vi "Periodic Tasks.vi"(8 "error in":errorcluster) -> ()   [LabVIEW 2019]
doc: "This VI runs in parallel to other tasks. It can contain as many user-defined periodic loops as you need. These can carry out PID or other sorts of timed response."
uses:
  <vilib>/Rock Robotics/WPI/Relay/WPI_RelayValue.ctl
  <vilib>/Rock Robotics/WPI/ThirdParty/Phoenix-LabVIEW/Motor Controller/Controls/CTRE_Phoenix_MotorControl_ControlMode.ctl
  <vilib>/Rock Robotics/WPI/Solenoid/WPI_SolenoidValue.ctl
  Driver Globals.vi
  <vilib>/Rock Robotics/WPI/Solenoid/WPI_SolenoidSetEnum.vi
panel:
  in  "Proportional":dbl
  in  "Integral":dbl
  in  "Derivative":dbl
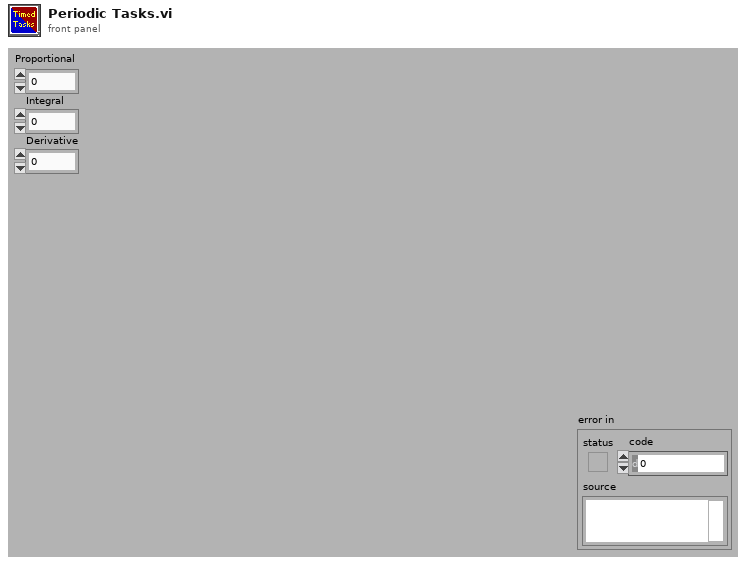
[diagram p1: front panel]
types:
  T1 = typedef "WPI_RelayValue.ctl" = enum16{"Off", "On", "Forward", "Reverse"}
  T2 = enum16{"DemandType_Neutral", "DemandType_AuxPID", "DemandType_ArbitraryFeedForward"}
  T3 = typedef "WPI_SolenoidValue.ctl" = enum16{"Off", "On", "Forward", "Reverse"}
  T4 = typedef "Color Sensor V3 DevRef.ctl" = cluster{"I2CDevRef":T5}
  T5 = typedef "WPI_I2CDevRef.ctl" = cluster{"DevStatus":errorcluster, "Device Address":u8, "Handle":i32, "I2C Bus":T6}
  T6 = typedef "i2c_bus.ctl" = enum16{"I2C On-Board", "I2C MXP", "Invalid"}
  T7 = typedef "WPI_EncoderDevRef.ctl" = cluster{"DevStatus":errorcluster, "EncoderIndex":T8, "CounterIndex":T9, "DistancePerCount":dbl, "Decoding Type":T10}
  T8 = typedef "FPGA_EncoderIdx.ctl" = enum8{"Enc 0", "Enc 1", "Enc 2", "Enc 3", "Enc 4", "Enc 5", "Enc 6", "Enc 7", "Invalid"}
  T9 = typedef "FPGA_CounterCtrSystemIndex.ctl" = enum8{"Ctr 0", "Ctr 1", "Ctr 2", "Ctr 3", "Ctr 4", "Ctr 5", "Ctr 6", "Ctr 7", "Invalid"}
  T10 = typedef "WPI_EncoderType.ctl" = enum16{"1x", "2x", "4x"}
  T11 = typedef "WPI_MotorControlDeviceRef.ctl" = cluster{"DeviceStatus":errorcluster, "Type":T12, "PWM":cluster{"PWM Channel":T13, "DeadBand":T14}, "CAN":cluster{"Device Number":u8, "SetOutput VI Ref":variant, "GetOutput VI Ref":variant, "Enable VI Ref":variant, "Disable VI Ref":variant, "Data":variant}, "Invert":bool, "DIO PWM":cluster{"PWM \"Enable\" Channel":T13, "DIOChannel":T15, "PWM Rate":dbl}}
  T12 = typedef "WPI_MotorControlType.ctl" = enum16{"PWM", "CAN", "DIO PWM"}
  T13 = typedef "FPGA_DIOPWMChannel.ctl" = enum8{"PWM 0", "PWM 1", "PWM 2", "PWM 3", "PWM 4", "PWM 5", "PWM 6", "PWM 7", "PWM 8", "PWM 9", "PWM MXP 0", "PWM MXP 1", "PWM MXP 2", "PWM MXP 3", "PWM MXP 4", "PWM MXP 5", "PWM MXP 6", "PWM MXP 7", "PWM MXP 8", "PWM MXP 9", "Invalid"}
  T14 = typedef "WPI_PWMDeadband.ctl" = cluster{"Name":string, "maxPositivePwm":i32, "minPositivePwm":i32, "centerPwm":i32, "maxNegativePwm":i32, "minNegativePwm":i32, "angularRange":u16}
  T15 = typedef "FPGA_DIOChannel.ctl" = enum8{"DIO 0", "DIO 1", "DIO 2", "DIO 3", "DIO 4", "DIO 5", "DIO 6", "DIO 7", "DIO 8", "DIO 9", "DIO MXP 0", "DIO MXP 1", "DIO MXP 2", "DIO MXP 3", "DIO MXP 4", "DIO MXP 5", "DIO MXP 6", "DIO MXP 7", "DIO MXP 8", "DIO MXP 9", "DIO MXP 10", "DIO MXP 11", "DIO MXP 12", "DIO MXP 13", "DIO MXP 14", "DIO MXP 15", "SPI Port CS1", "SPI Port CS2", "SPI Port CS3", "SPI Port MISO", "SPI Port MOSI", "Invalid"}
  T16 = typedef "WPI_AnalogChannelDevRef.ctl" = cluster{"DevStatus":errorcluster, "Analog Channel":T17}
  T17 = typedef "FPGA_AIChannel.ctl" = enum8{"AI 0", "AI 1", "AI 2", "AI 3", "AI MXP 0", "AI MXP 1", "AI MXP 2", "AI MXP 3", "Invalid"}
  T18 = typedef "WPI_SolenoidDevRef.ctl" = cluster{"DevStatus":errorcluster, "Pneumatics Control Module":u8, "Forward Solenoid Channel":T19, "Reverse Solenoid Channel":T19}
  T19 = typedef "WPI_SolenoidChannel.ctl" = enum8{"Solenoid 0", "Solenoid 1", "Solenoid 2", "Solenoid 3", "Solenoid 4", "Solenoid 5", "Solenoid 6", "Solenoid 7", "Invalid"}
  T20 = typedef "CTRE_Phoenix_MotorControl_ControlMode.ctl" = u16
  T21 = typedef "WPI_RelayDevRef.ctl" = cluster{"DevStatus":errorcluster, "Relay Channel":T22, "Relay Direction":T23}
  T22 = typedef "FPGA_DIORelayChannel.ctl" = enum8{"Relay 0", "Relay 1", "Relay 2", "Relay 3", "Invalid"}
  T23 = typedef "WPI_RelayDirection.ctl" = enum16{"Both directions", "Forward only", "Reverse only"}
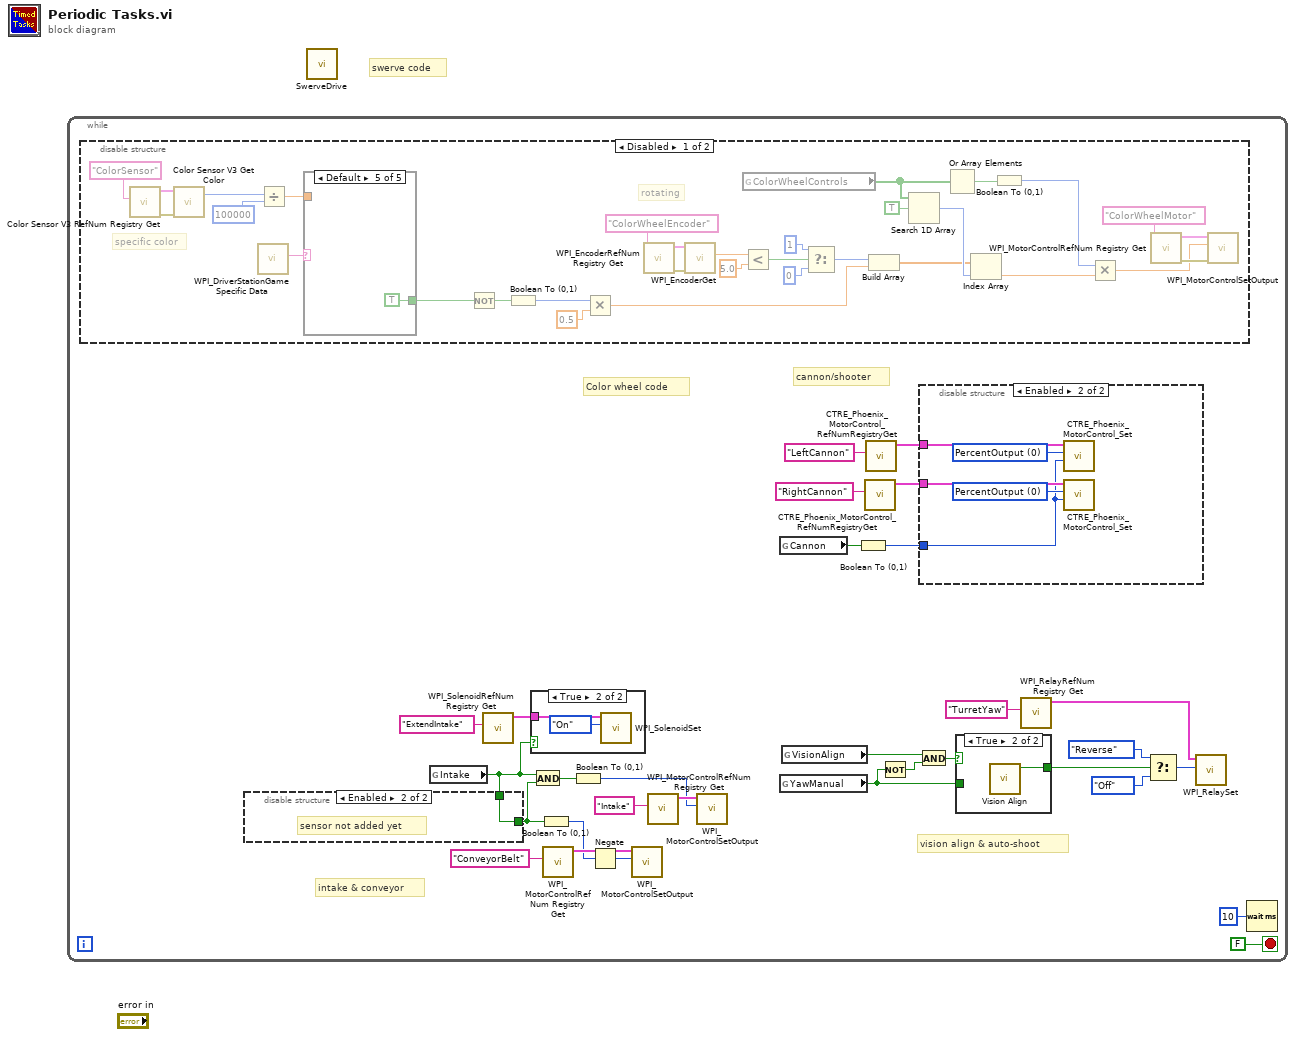
[diagram p0: block diagram]
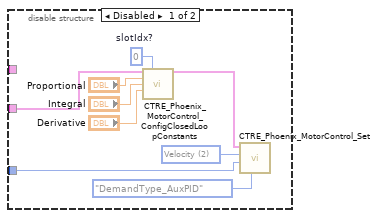
[diagram p2: hidden frame]
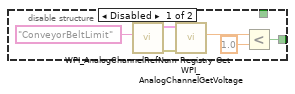
[diagram p3: hidden frame]
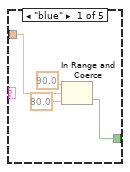
[diagram p5: hidden frame]
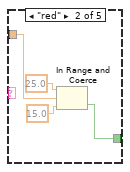
[diagram p6: hidden frame]
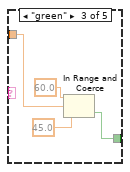
[diagram p7: hidden frame]
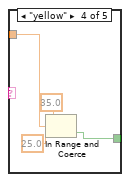
[diagram p8: hidden frame]
diagram:
  # "swerve code"
  n1 = while {
    stop <- FALSE stop-if-true
    # "intake & conveyor"
    # "vision align & auto-shoot"
    # "cannon/shooter"
    # "Color wheel code"
    n2 = disable-structure shown="Disabled" {
      frame Disabled {
        # "specific color"
        # "rotating"
        n3 = call <vilib>:"Color Sensor V3 RefNum Registry Get.vi"("refnum name"="ColorSensor") -> ("error out"=w81:errorcluster, "ColorSensorDevRef"=w80:T4)  [unwired: 9 in]
        n4 = call <vilib>:"Color Sensor V3 Get Color.vi"("error in (no error)"=w81, "ColorSensorDevRef"=w80) -> ("Color"=w78:u32)  [unwired: 6 in, 3 out]
        n5 = call <vilib>:"WPI_DriverStationGame Specific Data.vi"() -> ("Game Specific Data"=w82:string)  [unwired: 11 in]
        n6 = Divide(x=w78, y=u32 100000) -> (x/y=w76:dbl)
        n7 = case shown="Default" w82 {
          tunnel: w76 -> [w89 w93 w97 w101 _]
          tunnel: [w86 w90 w94 w98 TRUE] -> w54
          frame "blue" {
            n8 = In Range and Coerce(upper limit=90.0, x=w89, lower limit=80.0) -> (In Range?=w86:bool)  [unwired: 1 out]
          }
          frame "red" {
            n9 = In Range and Coerce(upper limit=25.0, x=w93, lower limit=15.0) -> (In Range?=w90:bool)  [unwired: 1 out]
          }
          frame "green" {
            n10 = In Range and Coerce(upper limit=60.0, x=w97, lower limit=45.0) -> (In Range?=w94:bool)  [unwired: 1 out]
          }
          frame "yellow" {
            n11 = In Range and Coerce(upper limit=35.0, x=w101, lower limit=25.0) -> (In Range?=w98:bool)  [unwired: 1 out]
          }
          frame Default {
          }
        }
        n12 = Not(x=w54) -> (.not. x?=w55:bool)
        n13 = Boolean To (0,1)(Boolean=w55) -> (0, 1=w56:i16)
        n14 = Multiply(x=w56, y=0.5) -> (x*y=w65:dbl)
        n15 = call <vilib>:"WPI_EncoderRefNum Registry Get.vi"("refnum name"="ColorWheelEncoder") -> ("error out"=w84:errorcluster, "EncoderDevRef"=w85:T7)  [unwired: 9 in]
        n16 = call <vilib>:"WPI_EncoderGet.vi"("error in (no error)"=w84, "EncoderDevRef"=w85) -> ("Distance"=w71:dbl)  [unwired: 4 in, 5 out]
        n17 = global read "Driver Globals.vi" "ColorWheelControls"() -> (w59:bool[])
        n18 = Less?(x=w71, y=5.0) -> (x < y?=w69:bool)
        n19 = Select(t=i16 1, s=w69, f=i16 0) -> (s? t:f=w66:i16)
        n20 = Build Array(w66, w65) -> (w61:dbl[])
        n21 = Search 1D Array(1D array=w59, element=TRUE) -> (index of element=w62:i32)  [unwired: 1 in]
        n22 = Or Array Elements(Boolean array=w59) -> (logical OR=w64:bool)
        n23 = Index Array(array=w61, index=w62) -> (element=w58:dbl)
        n24 = Boolean To (0,1)(Boolean=w64) -> (0, 1=w57:i16)
        n25 = Multiply(x=w57, y=w58) -> (x*y=w60:dbl)
        n26 = call <vilib>:"WPI_MotorControlRefNum Registry Get.vi"("refnum name"="ColorWheelMotor") -> ("error out"=w73:errorcluster, "MotorControlDevRef"=w74:T11)  [unwired: 9 in]
        n27 = call <vilib>:"WPI_MotorControlSetOutput.vi"("error in (no error)"=w73, "Output"=w60, "MotorControlDevRef"=w74) -> ()  [unwired: 6 in, 3 out]
      }
      frame Enabled {
      }
    }
    n28 = global read "Driver Globals.vi" "Intake"() -> (w13:bool)
    n29 = disable-structure shown="Enabled" {
      disable-tunnel: [w45 w51] -> w15
      disable-tunnel: w13 -> [_ w51]
      frame Disabled {
        n30 = call <vilib>:"WPI_AnalogChannelRefNum Registry Get.vi"("refnum name"="ConveyorBeltLimit") -> ("error out"=w50:errorcluster, "AIDeviceRef"=w49:T16)  [unwired: 9 in]
        n31 = call <vilib>:"WPI_AnalogChannelGetVoltage.vi"("error in (no error)"=w50, "AIDeviceRef"=w49) -> ("Voltage"=w47:dbl)  [unwired: 7 in, 2 out]
        n32 = Less?(x=w47, y=1.0) -> (x < y?=w45:bool)
      }
      frame Enabled {
        # "sensor not added yet"
      }
    }
    n33 = call <vilib>:"WPI_SolenoidRefNum Registry Get.vi"("refnum name"="ExtendIntake") -> ("SolenoidDevRef"=w18:T18)  [unwired: 9 in, 1 out]
    n34 = case shown="True" w13 {
      tunnel: w18 -> [_ w53]
      frame False {
      }
      frame True {
        n35 = call-poly <vilib>:"WPI_SolenoidSet.vi"("Value"=WPI_SolenoidValue."On", "SolenoidDevRef"=w53) -> ()  [unwired: 8 in, 2 out]
      }
    }
    n36 = And(x=w13, y=w15) -> (x .and. y?=w16:bool)
    n37 = Boolean To (0,1)(Boolean=w15) -> (0, 1=w8:i16)
    n38 = call <vilib>:"WPI_MotorControlRefNum Registry Get.vi"("refnum name"="ConveyorBelt") -> ("MotorControlDevRef"=w23:T11)  [unwired: 9 in, 1 out]
    n39 = Boolean To (0,1)(Boolean=w16) -> (0, 1=w14:i16)
    n40 = Negate(x=w8) -> (-x=w7:i16)
    n41 = call <vilib>:"WPI_MotorControlSetOutput.vi"("Output"=w7, "MotorControlDevRef"=w23) -> ()  [unwired: 7 in, 3 out]
    n42 = call <vilib>:"WPI_MotorControlRefNum Registry Get.vi"("refnum name"="Intake") -> ("MotorControlDevRef"=w28:T11)  [unwired: 9 in, 1 out]
    n43 = call <vilib>:"WPI_MotorControlSetOutput.vi"("Output"=w14, "MotorControlDevRef"=w28) -> ()  [unwired: 7 in, 3 out]
    n44 = global read "Driver Globals.vi" "Cannon"() -> (w20:bool)
    n45 = global read "Driver Globals.vi" "YawManual"() -> (w10:bool)
    n46 = global read "Driver Globals.vi" "VisionAlign"() -> (w11:bool)
    n47 = Boolean To (0,1)(Boolean=w20) -> (0, 1=w19:i16)
    n48 = call <vilib>:"CTRE_Phoenix_MotorControl_RefNumRegistryGet.vi"("refnum name"="RightCannon") -> ("PhoenixMotorControlDevRef"=w27:T11)  [unwired: 9 in, 1 out]
    n49 = call <vilib>:"CTRE_Phoenix_MotorControl_RefNumRegistryGet.vi"("refnum name"="LeftCannon") -> ("PhoenixMotorControlDevRef"=w1:T11)  [unwired: 9 in, 1 out]
    n50 = Not(x=w10) -> (.not. x?=w9:bool)
    n51 = And(x=w11, y=w9) -> (x .and. y?=w12:bool)
    n52 = disable-structure shown="Enabled" {
      disable-tunnel: w27 -> [w39 w44]
      disable-tunnel: w19 -> [w38 w40]
      disable-tunnel: w1 -> [_ w41]
      frame Disabled {
        w32 = 0  # slotIdx?
        w35 = T20 2 items=["PercentOutput"=0, "Position"=1, "Velocity"=2, "Current"=3, "Follower"=5, "MotionProfile"=6, "MotionMagic"=7, "MotionProfileArc"=10, "Disabled"=15] ("Control Mode")
        n53 = call <vilib>:"CTRE_Phoenix_MotorControl_ConfigClosedLoopConstants.vi"("PhoenixMotorControlDevRef"=w39, "slotIdx"=w32, "P"="Proportional", "I"="Integral", "D"="Derivative") -> ("PhoenixMotorControlDevRef"=w36:T11)  [unwired: 9 in, 1 out]
        n54 = call <vilib>:"CTRE_Phoenix_MotorControl_Set.vi"("DemandType"=T2."DemandType_AuxPID", "Output"=w38, "Control Mode"=w35, "PhoenixMotorControlDevRef"=w36) -> ()  [unwired: 6 in, 2 out]
      }
      frame Enabled {
        w42 = T20 0 items=["PercentOutput"=0, "Position"=1, "Velocity"=2, "Current"=3, "Follower"=5, "MotionProfile"=6, "MotionMagic"=7, "MotionProfileArc"=10, "Disabled"=15] ("Control Mode")
        w43 = T20 0 items=["PercentOutput"=0, "Position"=1, "Velocity"=2, "Current"=3, "Follower"=5, "MotionProfile"=6, "MotionMagic"=7, "MotionProfileArc"=10, "Disabled"=15] ("Control Mode")
        n55 = call <vilib>:"CTRE_Phoenix_MotorControl_Set.vi"("Output"=w40, "Control Mode"=w42, "PhoenixMotorControlDevRef"=w41) -> ()  [unwired: 7 in, 2 out]
        n56 = call <vilib>:"CTRE_Phoenix_MotorControl_Set.vi"("Output"=w40, "Control Mode"=w43, "PhoenixMotorControlDevRef"=w44) -> ()  [unwired: 7 in, 2 out]
      }
    }
    n57 = case shown="True" w12 {
      tunnel: w10 -> [w103 _]
      tunnel: [w103 w104] -> w6
      frame False {
      }
      frame True {
        n58 = call "Vision Align.vi"() -> ("YawOut"=w104:bool)  [unwired: 11 in]
      }
    }
    n59 = call <vilib>:"WPI_RelayRefNum Registry Get.vi"("refnum name"="TurretYaw") -> ("RelayDevRef"=w22:T21)  [unwired: 9 in, 1 out]
    n60 = Select(t=WPI_RelayValue."Reverse" ("RelayValue"), s=w6, f=WPI_RelayValue."Off" ("RelayValue")) -> (s? t:f=w4:T1)
    n61 = call <vilib>:"WPI_RelaySet.vi"("RelayValue"=w4, "RelayDevRef"=w22) -> ()  [unwired: 8 in, 2 out]
    n62 = Wait (ms)(milliseconds to wait=u32 10) -> ()  [unwired: 1 out]
  }
  n63 = call "SwerveDrive.vi"() -> ()  [unwired: 12 in]
